vi "Initialise.vi"(8 "error in (no error)":errorcluster, 10 "Instrument Ref":string, 11 "Hioki9002 Switch":refnum<class "Hioki9002.lvclass">) -> (0 "error out":errorcluster, 3 "Hioki9002 Switch":refnum<class "Hioki9002.lvclass">)   [LabVIEW 2019, in "Concrete.lvlib" / "Hioki9002.lvclass"]
uses:
  Hioki9002.lvclass
  Hioki9002.lvclass/Hioki9002.ctl
  <instrlib>/HIOKI SW100X Series/Public/_Initialize/Initialize_USB.vi
  Harware Abstraction/Switch/Switch.lvclass
  <instrlib>/HIOKI SW100X Series/HIOKI SW100X Series.lvlib
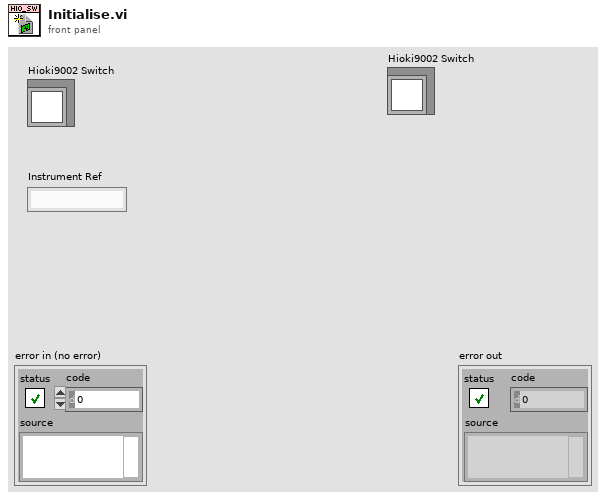
[diagram p1: front panel]
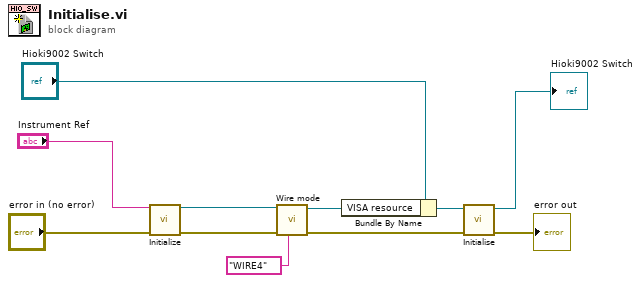
[diagram p0: block diagram]
diagram:
  n1 = call-poly <instrlib>:"Initialize.vi"("VISA resource name"="Instrument Ref", "error in (no error)"="error in (no error)") -> ("VISA resource name out"=w1:refnum<visa-resource-name>, "error out"=w2:errorcluster)  [unwired: 11 in, 1 out]
  n2 = call <instrlib>:"Wire mode.vi"("Connection method"="WIRE4", "error in"=w2, "VISA resource name"=w1) -> ("error out"=w9:errorcluster, "VISA resource name out"=w7:refnum<visa-resource-name>)  [unwired: 6 in, 1 out]
  n3 = Bundle By Name(cluster="Hioki9002 Switch", "VISA resource"=w7) -> (w8:refnum<class "Hioki9002.lvclass">)
  n4 = call-parent "Initialise.vi"("error in (no error)"=w9, "Instrument in"=w8) -> ("error out"=→"error out":errorcluster, "Instrument out"=→"Hioki9002 Switch":refnum<class "Hioki9002.lvclass">)  [unwired: 8 in]
